vi "Flow_velocity_process.vi"(3 "error in":errorcluster) -> (0 "error out":errorcluster)   [LabVIEW 2013]
uses:
  <vilib>/Analysis/NI_AALPro.lvlib
  <vilib>/Analysis/_algsub.llb/Real Vector Norm.vi
panel:
  in  "NSensors":i32
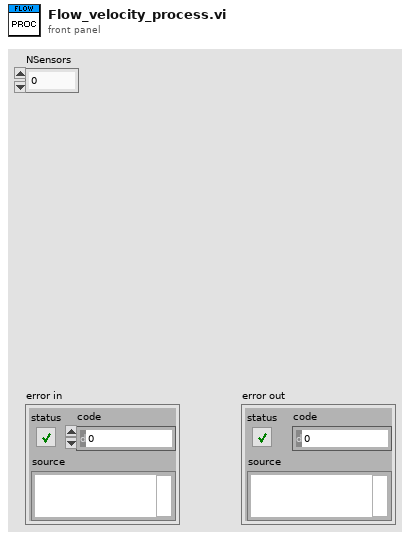
[diagram p1: front panel]
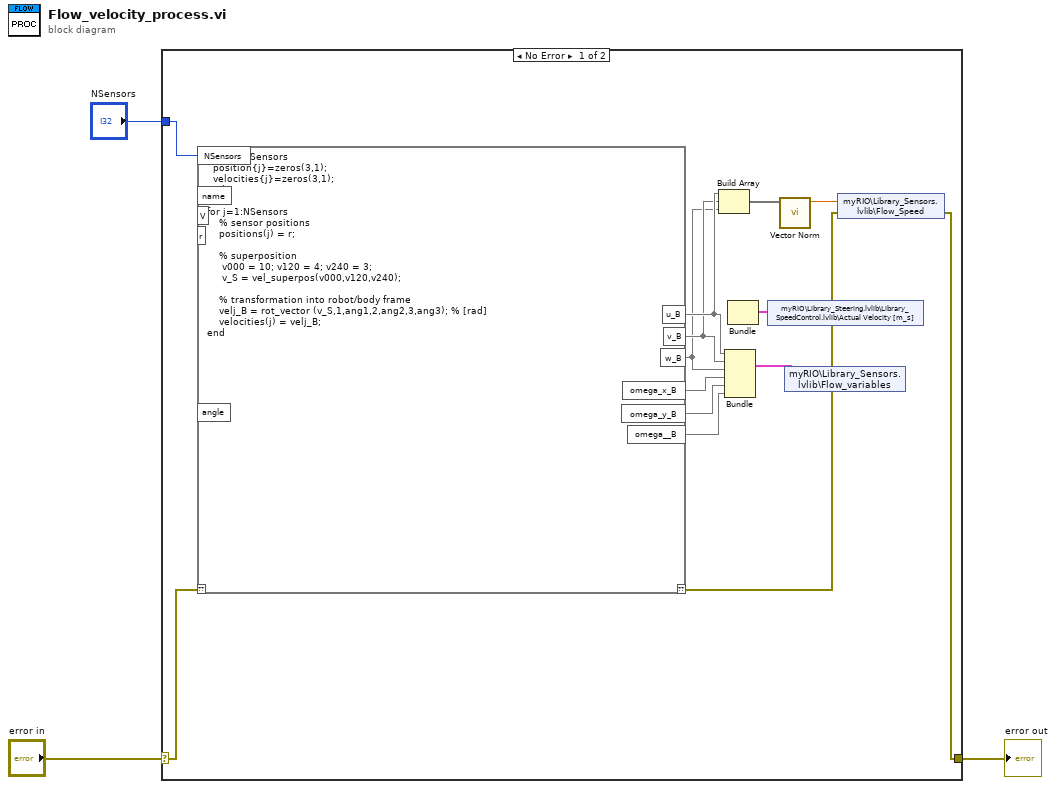
[diagram p0: block diagram]
diagram:
  n1 = case shown="No Error" "error in" {
    selector: "error in" -> [w7 w18]
    tunnel: [w5 w18] -> w2
    tunnel: "NSensors" -> [w13 _]
    frame No Error {
      n2 = mathscript code="for j=1:NSensors\n  position{j}=zeros(3,1);\n  velocities{j}=zeros(3,1);\nend\n\nfor j=1:NSensors\n    % sensor positions\n    positions(j) = r;\n\n    % superposition\n     v000 = 10; v120 = 4; v240 = 3;\n     v_S = vel_superpos(v000,v120,v240);\n\n    % transformation into robot/body frame\n    velj_B = rot_vector (v_S,1,ang1,2,ang2,3,ang3); % [rad]\n    velocities(j) = velj_B;\nend"("??"=w7, "NSensors"=w13) -> ("??"=w6:errorcluster, "u_B"=w12, "v_B"=w11, "w_B"=w10, "omega_x_B"=w16, "omega_y_B"=w15, "omega__B"=w14)  [unwired: 4 in]
      n3 = Build Array(w12, w11, w10) -> (w9:void[])
      n4 = Bundle(w12, w11, w10, w16, w15, w14) -> (w8:cluster{void, void, void, void, void, void})  [unwired: 1 in]
      n5 = Bundle() -> (w4:cluster{void, void, void})  [unwired: 4 in]
      n6 = shared-variable "myRIO\\Library_Steering.lvlib\\Library_SpeedControl.lvlib\\Actual Velocity [m_s]"(w4) -> ()  [unwired: 1 in, 1 out]
      n7 = call-poly <vilib>:"Vector Norm.vi"("Input Vector"=w9) -> ("norm"=w17:dbl)  [unwired: 9 in, 1 out]
      n8 = shared-variable "myRIO\\Library_Sensors.lvlib\\Flow_variables"(w8) -> ()  [unwired: 1 in, 1 out]
      n9 = shared-variable "myRIO\\Library_Sensors.lvlib\\Flow_Speed"(w17, error in=w6) -> (error out=w5:errorcluster)
    }
    frame Error {
    }
  }
  "error out" <- w2
